vi "Set TestMode.vi"(8 "error in (no error)":errorcluster, 10 "Test Mode":bool, 11 "RTL-SDR in":refnum<class "RTL-SDR.lvclass">) -> (0 "error out":errorcluster, 1 "function return":i32, 3 "RTL-SDR out":refnum<class "RTL-SDR.lvclass">)   [LabVIEW 2015, in "RTL-SDR.lvclass"]
doc: "Created IvanLis by LabVIEW Portal\nProfile: http://labviewportal.org/memberlist.php?mode=viewprofile&u=987\neMail: IvanLisanov@gMail.com\nTelegram: https://t.me/IvanLis"
uses:
  RTL-SDR.lvclass
  RTL-SDR.lvclass/RTL-SDR.ctl
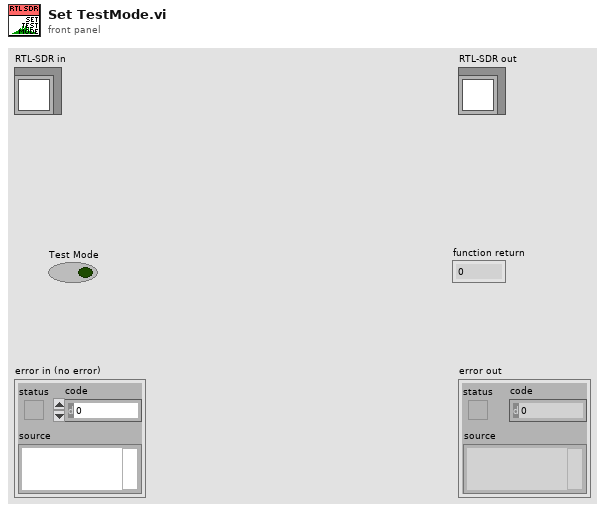
[diagram p1: front panel]
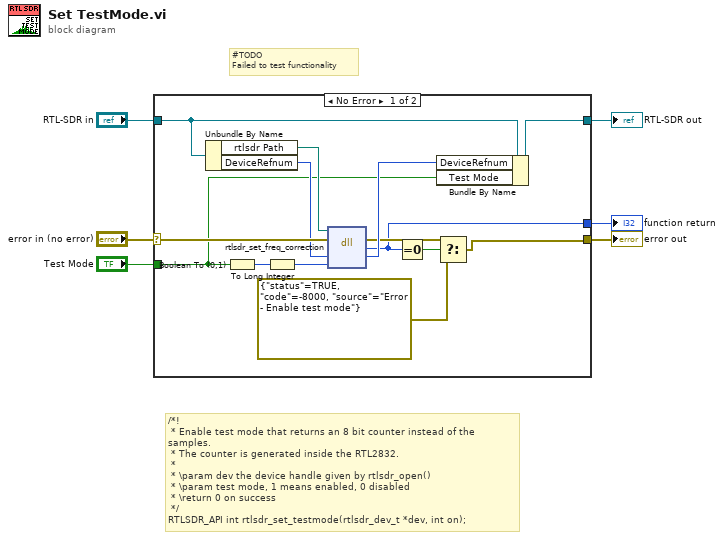
[diagram p0: block diagram]
diagram:
  # "#TODO\nFailed to test functionality"
  # "/*!\n * Enable test mode that returns an 8 bit counter instead of the samples.\n * The counter is generated inside the RTL2832.\n *\n * \\param dev the device handle given by rtlsdr_open()\n * \\param test mode, 1 means enabled, 0 disabled\n * \\return 0 on success\n */\nRTLSDR_API int rtlsdr_set_testmode(rtlsdr_dev_t *dev, int on);"
  n1 = case shown="No Error" "error in (no error)" {
    selector: "error in (no error)" -> [w20 w22]
    tunnel: [w11 w22] -> w5
    tunnel: [w18 w21] -> w3
    tunnel: "RTL-SDR in" -> [w19 w21]
    tunnel: [w12 _] -> w2
    tunnel: "Test Mode" -> [w8 _]
    frame No Error {
      n2 = Unbundle By Name(w19) -> ("rtlsdr Path"=w15:path, "DeviceRefnum"=w17:u64)
      n3 = Boolean To (0,1)(Boolean=w8) -> (0, 1=w9:i16)
      n4 = To Long Integer(number=w9) -> (32bit integer=w7:i32)
      n5 = dll-call lib="C:/Users/Ivan/Desktop/D-23-09-24 (RTL-SDR)/Project (Pelleng-SDR)/RTL-SDR Class/dll/rtlsdr.*" fn="rtlsdr_set_freq_correction"(path in=w15, error in=w20, "DeviceRefnum"=w17, "Frequency Correction (ppm)"=w7) -> (error out=w13:errorcluster, "return type"=w12:i32, "DeviceRefnum"=w16:u64)  [unwired: 2 in, 1 out]
      n6 = Equal To 0?(x=w12) -> (x = 0?=w14:bool)
      n7 = Bundle By Name(cluster=w19, "DeviceRefnum"=w16, "Test Mode"=w8) -> (w18:refnum<class "RTL-SDR.lvclass">)
      n8 = Select(t=w13, s=w14, f=errorcluster {"status"=TRUE, "code"=-8000, "source"="Error - Enable test mode"} ("error out")) -> (s? t:f=w11:errorcluster)
    }
    frame Error {
    }
  }
  "error out" <- w5
  "RTL-SDR out" <- w3
  "function return" <- w2
